vi "LED 7segment Example 2 Some text.vi"() -> ()   [LabVIEW 2014]
doc: "Light up 7segment LED."
panel:
  out "error out":errorcluster
  in  "error in":errorcluster
  # "+----------+\n|                |\n|                |\n|                |\n+----------+\n|                |\n|                |\n|                |\n+----------+ +"
  # "pin 9"
  # "pin 8"
  # "pin 10"
  # "pin 7"
  # "pin 6"
  # "pin 3"
  # "pin 4"
  # "pin 2"
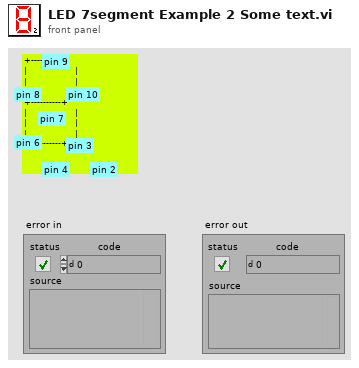
[diagram p1: front panel]
types:
  T1 = enum16{"nothing", "0", "1", "2", "3", "4", "5", "6", "7", "8", "9", "A", "B", "C", "D", "E", "F", "J", "L", "O", "P", "S", "U", "russian N", "russian U"}[]
  T2 = enum16{"nothing", "0", "1", "2", "3", "4", "5", "6", "7", "8", "9", "A", "B", "C", "D", "E", "F", "J", "L", "O", "P", "S", "U", "russian N", "russian U"}
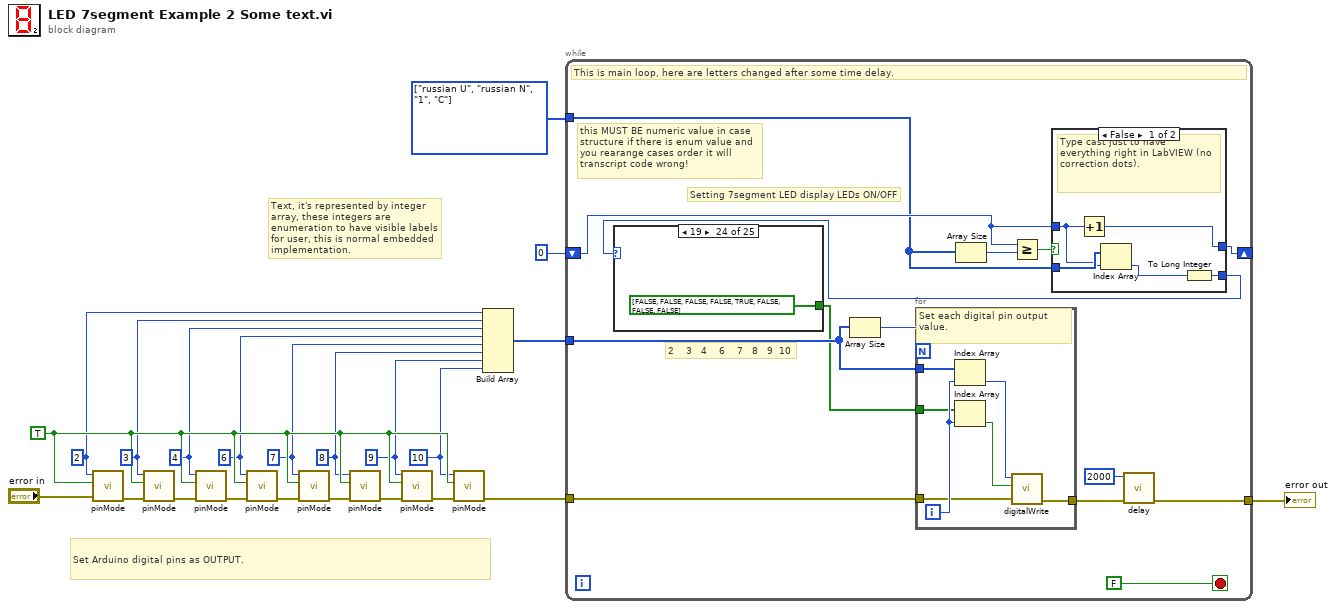
[diagram p0: block diagram]
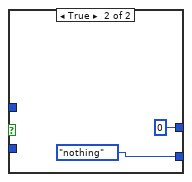
[diagram p2: hidden frame]
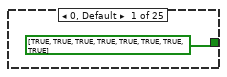
[diagram p3: hidden frame]
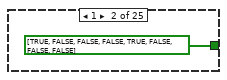
[diagram p4: hidden frame]
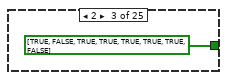
[diagram p5: hidden frame]
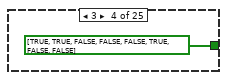
[diagram p6: hidden frame]
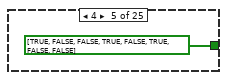
[diagram p7: hidden frame]
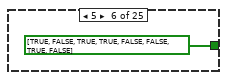
[diagram p8: hidden frame]
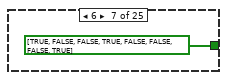
[diagram p9: hidden frame]
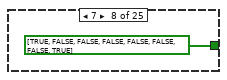
[diagram p10: hidden frame]
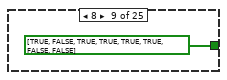
[diagram p11: hidden frame]
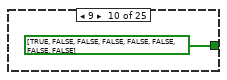
[diagram p12: hidden frame]
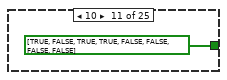
[diagram p13: hidden frame]
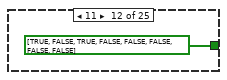
[diagram p14: hidden frame]
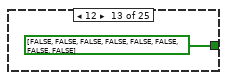
[diagram p15: hidden frame]
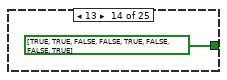
[diagram p16: hidden frame]
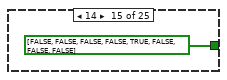
[diagram p17: hidden frame]
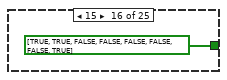
[diagram p18: hidden frame]
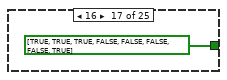
[diagram p19: hidden frame]
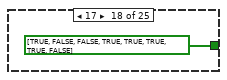
[diagram p20: hidden frame]
diagram:
  w2 = T1 [enum."russian U", enum."russian N", enum."1", enum."C"] items=["nothing", "0", "1", "2", "3", "4", "5", "6", "7", "8", "9", "A", "B", "C", "D", "E", "F", "J", "L", "O", "P", "S", "U", "russian N", "russian U"]
  w4 = 10 ("pin number")
  w5 = 9 ("pin number")
  w6 = 8 ("pin number")
  w7 = 7 ("pin number")
  w8 = 6 ("pin number")
  w9 = 4 ("pin number")
  w10 = 3 ("pin number")
  w11 = 2 ("pin number")
  w14 = TRUE ("output?")
  # "Text, it's represented by integer array, these integers are enumeration to have visible labels for user, this is normal embedded implementation."
  # "Set Arduino digital pins as OUTPUT."
  n1 = call <vilib>:"pinMode.vi"("Error In"="error in", "output?"=w14, "pin number"=w11) -> ("Error Out"=w21:errorcluster)  [unwired: 8 in]
  n2 = call <vilib>:"pinMode.vi"("Error In"=w21, "output?"=w14, "pin number"=w10) -> ("Error Out"=w15:errorcluster)  [unwired: 8 in]
  n3 = call <vilib>:"pinMode.vi"("Error In"=w15, "output?"=w14, "pin number"=w9) -> ("Error Out"=w20:errorcluster)  [unwired: 8 in]
  n4 = call <vilib>:"pinMode.vi"("Error In"=w20, "output?"=w14, "pin number"=w8) -> ("Error Out"=w19:errorcluster)  [unwired: 8 in]
  n5 = call <vilib>:"pinMode.vi"("Error In"=w19, "output?"=w14, "pin number"=w7) -> ("Error Out"=w17:errorcluster)  [unwired: 8 in]
  n6 = call <vilib>:"pinMode.vi"("Error In"=w17, "output?"=w14, "pin number"=w6) -> ("Error Out"=w16:errorcluster)  [unwired: 8 in]
  n7 = call <vilib>:"pinMode.vi"("Error In"=w16, "output?"=w14, "pin number"=w5) -> ("Error Out"=w18:errorcluster)  [unwired: 8 in]
  n8 = call <vilib>:"pinMode.vi"("Error In"=w18, "output?"=w14, "pin number"=w4) -> ("Error Out"=w12:errorcluster)  [unwired: 8 in]
  n9 = Build Array(w11, w10, w9, w8, w7, w6, w5, w4) -> (w3:i32[])
  n10 = while {
    tunnel: [w35] -> w22
    tunnel: w12 -> [w32]
    tunnel: w3 -> [w33]
    shift-right: [w27] -> _
    shift-left: 0 ("pin number") -> [w26]
    tunnel: w2 -> [w23]
    stop <- FALSE stop-if-true
    # "this MUST BE numeric value in case structure if there is enum value and you rearange cases order it will transcript code wrong!"
    # "Setting 7segment LED display LEDs ON/OFF"
    # "2    3   4    6    7   8   9  10"
    # "This is main loop, here are letters changed after some time delay."
    n11 = Array Size(array=w33) -> (size(s)=w29:i32)
    n12 = Array Size(array=w23) -> (size(s)=w24:i32)
    n13 = Greater Or Equal?(x=w26, y=w24) -> (x >= y?=w28:bool)
    n14 = case shown="False" w28 {
      tunnel: [w41 0] -> w27
      tunnel: w26 -> [w39 _]
      tunnel: w23 -> [w40 _]
      tunnel: [w37 T2."nothing"] -> w25
      frame False {
        # "Type cast just to have everything right in LabVIEW (no correction dots)."
        n15 = Increment(x=w39) -> (x+1=w41:i32)
        n16 = Index Array(array=w40, index=w39) -> (element=w38:T2)
        n17 = To Long Integer(number=w38) -> (32bit integer=w37:i32)
      }
      frame True {
      }
    }
    n18 = case shown="19" w25 {
      tunnel: [bool[] [TRUE, TRUE, TRUE, TRUE, TRUE, TRUE, TRUE, TRUE] bool[] [TRUE, FALSE, FALSE, FALSE, TRUE, FALSE, FALSE, FALSE] bool[] [TRUE, FALSE, TRUE, TRUE, TRUE, TRUE, TRUE, FALSE] bool[] [TRUE, TRUE, FALSE, FALSE, FALSE, TRUE, FALSE, FALSE] bool[] [TRUE, FALSE, FALSE, TRUE, FALSE, TRUE, FALSE, FALSE] bool[] [TRUE, FALSE, TRUE, TRUE, FALSE, FALSE, TRUE, FALSE] bool[] [TRUE, FALSE, FALSE, TRUE, FALSE, FALSE, FALSE, TRUE] bool[] [TRUE, FALSE, FALSE, FALSE, FALSE, FALSE, FALSE, TRUE] bool[] [TRUE, FALSE, TRUE, TRUE, TRUE, TRUE, FALSE, FALSE] bool[] [TRUE, FALSE, FALSE, FALSE, FALSE, FALSE, FALSE, FALSE] bool[] [TRUE, FALSE, TRUE, TRUE, FALSE, FALSE, FALSE, FALSE] bool[] [TRUE, FALSE, TRUE, FALSE, FALSE, FALSE, FALSE, FALSE] bool[] [FALSE, FALSE, FALSE, FALSE, FALSE, FALSE, FALSE, FALSE] bool[] [TRUE, TRUE, FALSE, FALSE, TRUE, FALSE, FALSE, TRUE] bool[] [FALSE, FALSE, FALSE, FALSE, TRUE, FALSE, FALSE, FALSE] bool[] [TRUE, TRUE, FALSE, FALSE, FALSE, FALSE, FALSE, TRUE] bool[] [TRUE, TRUE, TRUE, FALSE, FALSE, FALSE, FALSE, TRUE] bool[] [TRUE, FALSE, FALSE, TRUE, TRUE, TRUE, TRUE, FALSE] bool[] [FALSE, FALSE, FALSE, TRUE, FALSE, FALSE, FALSE, FALSE] bool[] [TRUE, FALSE, TRUE, FALSE, FALSE, FALSE, TRUE, FALSE] bool[] [TRUE, FALSE, FALSE, FALSE, TRUE, FALSE, TRUE, FALSE] bool[] [TRUE, TRUE, TRUE, FALSE, FALSE, FALSE, FALSE, FALSE] bool[] [TRUE, FALSE, FALSE, TRUE, FALSE, FALSE, FALSE, TRUE] bool[] [FALSE, FALSE, FALSE, FALSE, TRUE, FALSE, FALSE, FALSE] bool[] [TRUE, TRUE, FALSE, FALSE, TRUE, FALSE, TRUE, TRUE]] -> w30
      frame 0, Default {
      }
      frame 1 {
      }
      frame 2 {
      }
      frame 3 {
      }
      frame 4 {
      }
      frame 5 {
      }
      frame 6 {
      }
      frame 7 {
      }
      frame 8 {
      }
      frame 9 {
      }
      frame 10 {
      }
      frame 11 {
      }
      frame 12 {
      }
      frame 13 {
      }
      frame 14 {
      }
      frame 15 {
      }
      frame 16 {
      }
      frame 17 {
      }
      frame 24 {
      }
      frame 23 {
      }
      frame 22 {
      }
      frame 20 {
      }
      frame 21 {
      }
      frame 19 {
      }
      frame 18 {
      }
    }
    n19 = for {
      N: w29 -> [_]
      tunnel: w33 -> [w50]
      tunnel: w32 -> [w47]
      tunnel: [w46] -> w31
      tunnel: w30 -> [w45]
      i -> [w48]
      # "Set each digital pin output value."
      n20 = Index Array(array=w50, index=w48) -> (element=w49:i32)
      n21 = Index Array(array=w45, index=w48) -> (element=w44:bool)
      n22 = call <vilib>:"digitalWrite.vi"("Error In"=w47, "value"=w44, "pin number"=w49) -> ("Error Out"=w46:errorcluster)  [unwired: 8 in]
    }
    n23 = call <vilib>:"delay.vi"("Error In"=w31, "time (ms)"=2000) -> ("Error Out"=w35:errorcluster)  [unwired: 9 in]
  }
  "error out" <- w22
